vi "Vector Cal.vi"() -> ()   [LabVIEW 2016]
uses:
  <vilib>/Utility/file.llb/Read Delimited Spreadsheet (DBL).vi
panel:
  out "travel rotation\ndegrees":dbl[](array[numeric])
  out "Turning Angle (deg)":dbl[](array[numeric])
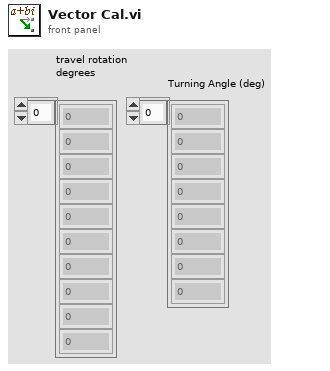
[diagram p1: front panel]
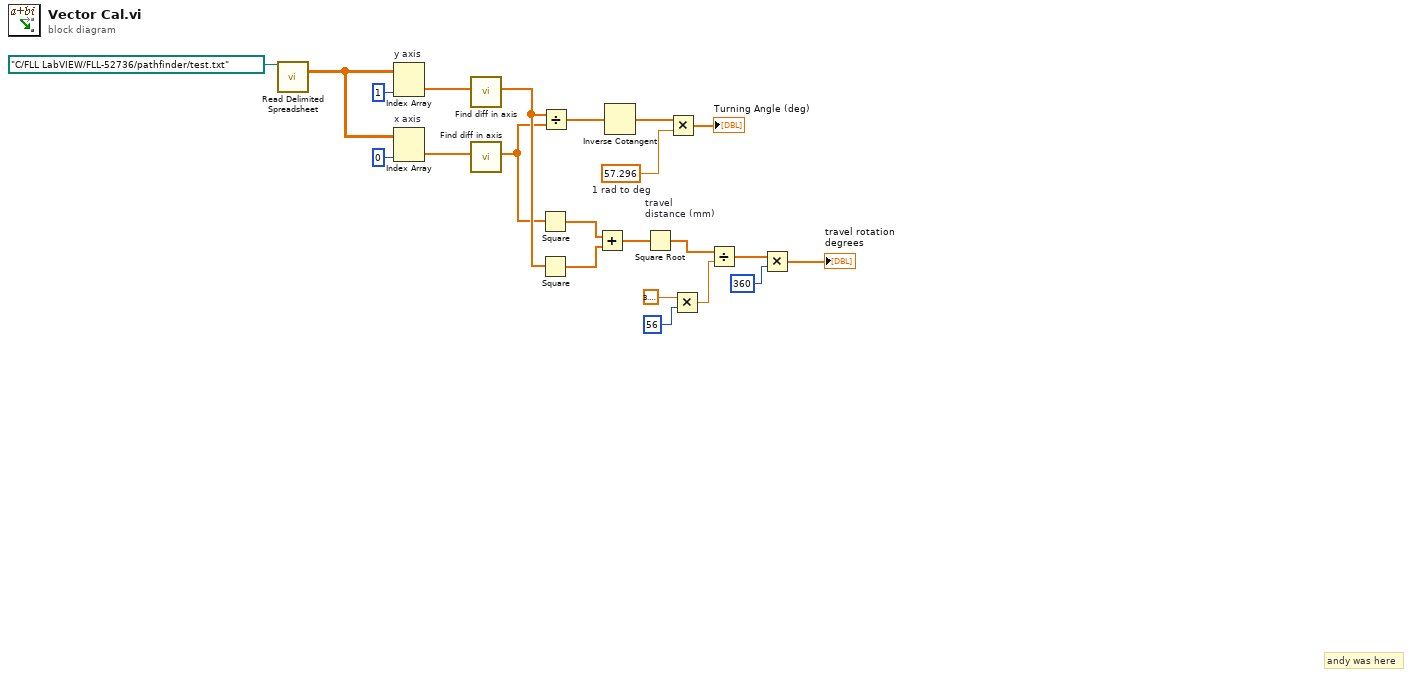
[diagram p0: block diagram]
diagram:
  w14 = 57.296  # 1 rad to deg
  # "andy was here"
  n1 = call-poly <vilib>:"Read Delimited Spreadsheet.vi"("file path (dialog if empty)"=path "C:/FLL LabVIEW/FLL-52736/pathfinder/test.txt") -> ("all rows"=w19:dbl[][])  [unwired: 9 in, 5 out]
  n2 = Index Array "y axis"(array=w19, index (col)=1 ("disabled index (col)")) -> (element=w18:dbl[])  [unwired: 1 in]
  n3 = Index Array "x axis"(array=w19, index (col)=0 ("disabled index (col)")) -> (element=w17:dbl[])  [unwired: 1 in]
  n4 = call "Find diff in axis.vi"("array"=w18) -> ("x,y2 - x,y1"=w12:dbl[])  [unwired: 10 in]
  n5 = call "Find diff in axis.vi"("array"=w17) -> ("x,y2 - x,y1"=w11:dbl[])  [unwired: 10 in]
  n6 = Square(x=w11) -> (x^2=w10:dbl[])
  n7 = Square(x=w12) -> (x^2=w9:dbl[])
  n8 = Divide(x=w12, y=w11) -> (x/y=w16:dbl[])
  n9 = Add(x=w10, y=w9) -> (x+y=w8:dbl[])
  n10 = Inverse Cotangent(1:w16) -> (0:w15:dbl[])
  n11 = Square Root "travel\ndistance (mm)"(x=w8) -> (sqrt(x)=w7:dbl[])
  n12 = Multiply(x=w15, y=w14) -> (x*y=→"Turning Angle (deg)":dbl[])
  n13 = Multiply(x=3.141592653589793, y=56) -> (x*y=w4:dbl)
  n14 = Divide(x=w7, y=w4) -> (x/y=w3:dbl[])
  n15 = Multiply(x=w3, y=360) -> (x*y=→"travel rotation\ndegrees":dbl[])
